vi "Play Wav.vi"(1 "path":path) -> (0 "is playing?":bool)   [LabVIEW 2016, in "Common.lvlib"]
uses:
  <userlib>/Common Components/Common/Common.lvlib
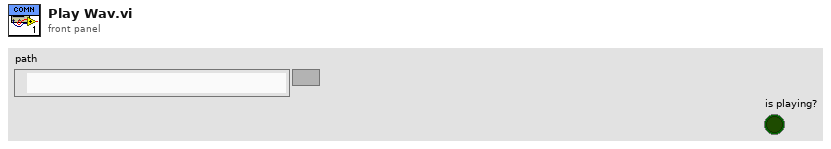
[diagram p1: front panel]
types:
  T1 = typedef "Sound Output Task ID.ctl" = u32
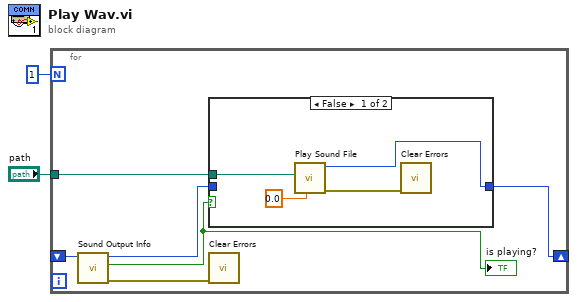
[diagram p0: block diagram]
diagram:
  n1 = for {
    N: 1 -> [_]
    tunnel: "path" -> [w8]
    shift-right: [w7] -> _
    shift-left: _ -> [w6]
    n2 = call <vilib>:"Sound Output Info.vi"("task ID"=w6) -> ("error out"=w3:errorcluster, "is playing?"=w5:bool, "task ID out"=w4:T1)  [unwired: 7 in, 1 out]
    "is playing?" <- w5
    n3 = case shown="False" w5 {
      tunnel: w8 -> [w12 _]
      tunnel: [w10 w13] -> w7
      tunnel: w4 -> [_ w13]
      frame False {
        n4 = call <vilib>:"Play Sound File.vi"("timeout (sec)"=0.0, "path"=w12) -> ("error out"=w9:errorcluster, "task ID"=w10:T1)  [unwired: 8 in]
        n5 = call <vilib>:"Clear Errors.vi"("error in (no error)"=w9) -> ()  [unwired: 5 in, 2 out]
      }
      frame True {
      }
    }
    n6 = call <vilib>:"Clear Errors.vi"("error in (no error)"=w3) -> ()  [unwired: 5 in, 2 out]
  }
